vi "CPC_Surveillence_App_Overlay.vi"() -> ()   [LabVIEW 2013]
uses:
  <vilib>/userdefined/High Color/IMAQdx.ctl
  <vilib>/vision/driver/IMAQdx.llb/IMAQdx Buffer Number Mode.ctl
  <vilib>/vision/driver/NI_Vision_Acquisition_Software.lvlib
  <vilib>/vision/NI_Vision_Development_Module.lvlib
panel:
  in  "Cam1":T1
  in  "Cam0":T1
  out "Recording 2":bool
  out "Recording 2":dbl
  out "Cam 1":T2(plugin-control)
  out "Motion Detection 2":bool
  out "No Motion 2":bool caption="Time has Elapsed"
  out "Cam 0":T2(plugin-control)
  out "Motion Detection":bool
  out "No Motion":bool caption="Time has Elapsed"
  in  "Root Directory":path
  in  "Frames/s":u32=30
  out "Recording":bool
  out "Frames/s":dbl
  in  "Exit App":bool
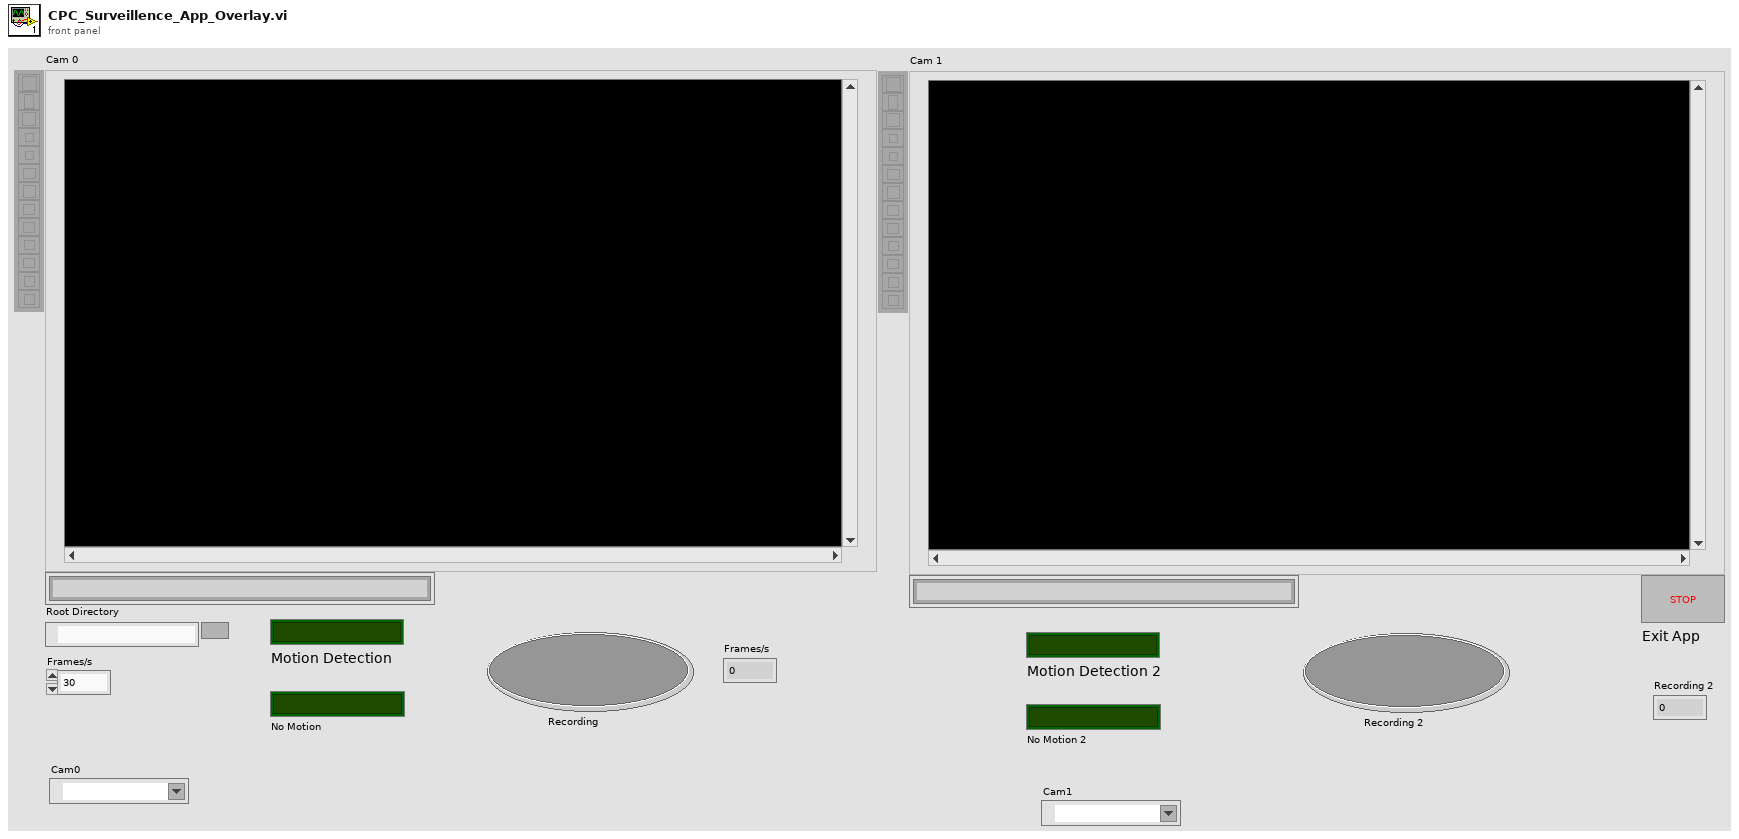
[diagram p1: front panel]
types:
  T1 = typedef "IMAQdx.ctl" = refnum<k21>
  T2 = typedef "IMAQ Image.ctl" = refnum<image>
  T3 = enum8{"Enabled", "Disabled", "Disabled and Grayed Out"}
  T4 = cluster{"Desired Font (Application)":enum16{"User-specified Font", "Application Font", "System Font", "Dialog Font"}, "[User-specified Font]":cluster{"Font Name":string, "Size":i16, "Strikeout?":bool, "Italic?":bool, "Underline?":bool, "Outline?":bool, "Shadow?":bool, "Bold?":bool, "Rotation Angle":dbl}, "Horizontal Alignment":i16, "Vertical Alignment":i16}
  T5 = typedef "NI_Vision_Acquisition_Software.lvlib/IMAQdx Buffer Number Mode.ctl" = enum32{"Next", "Last", "Buffer Number"}
  T6 = typedef "IMAQ AVI2 Refnum.ctl" = refnum<k20>
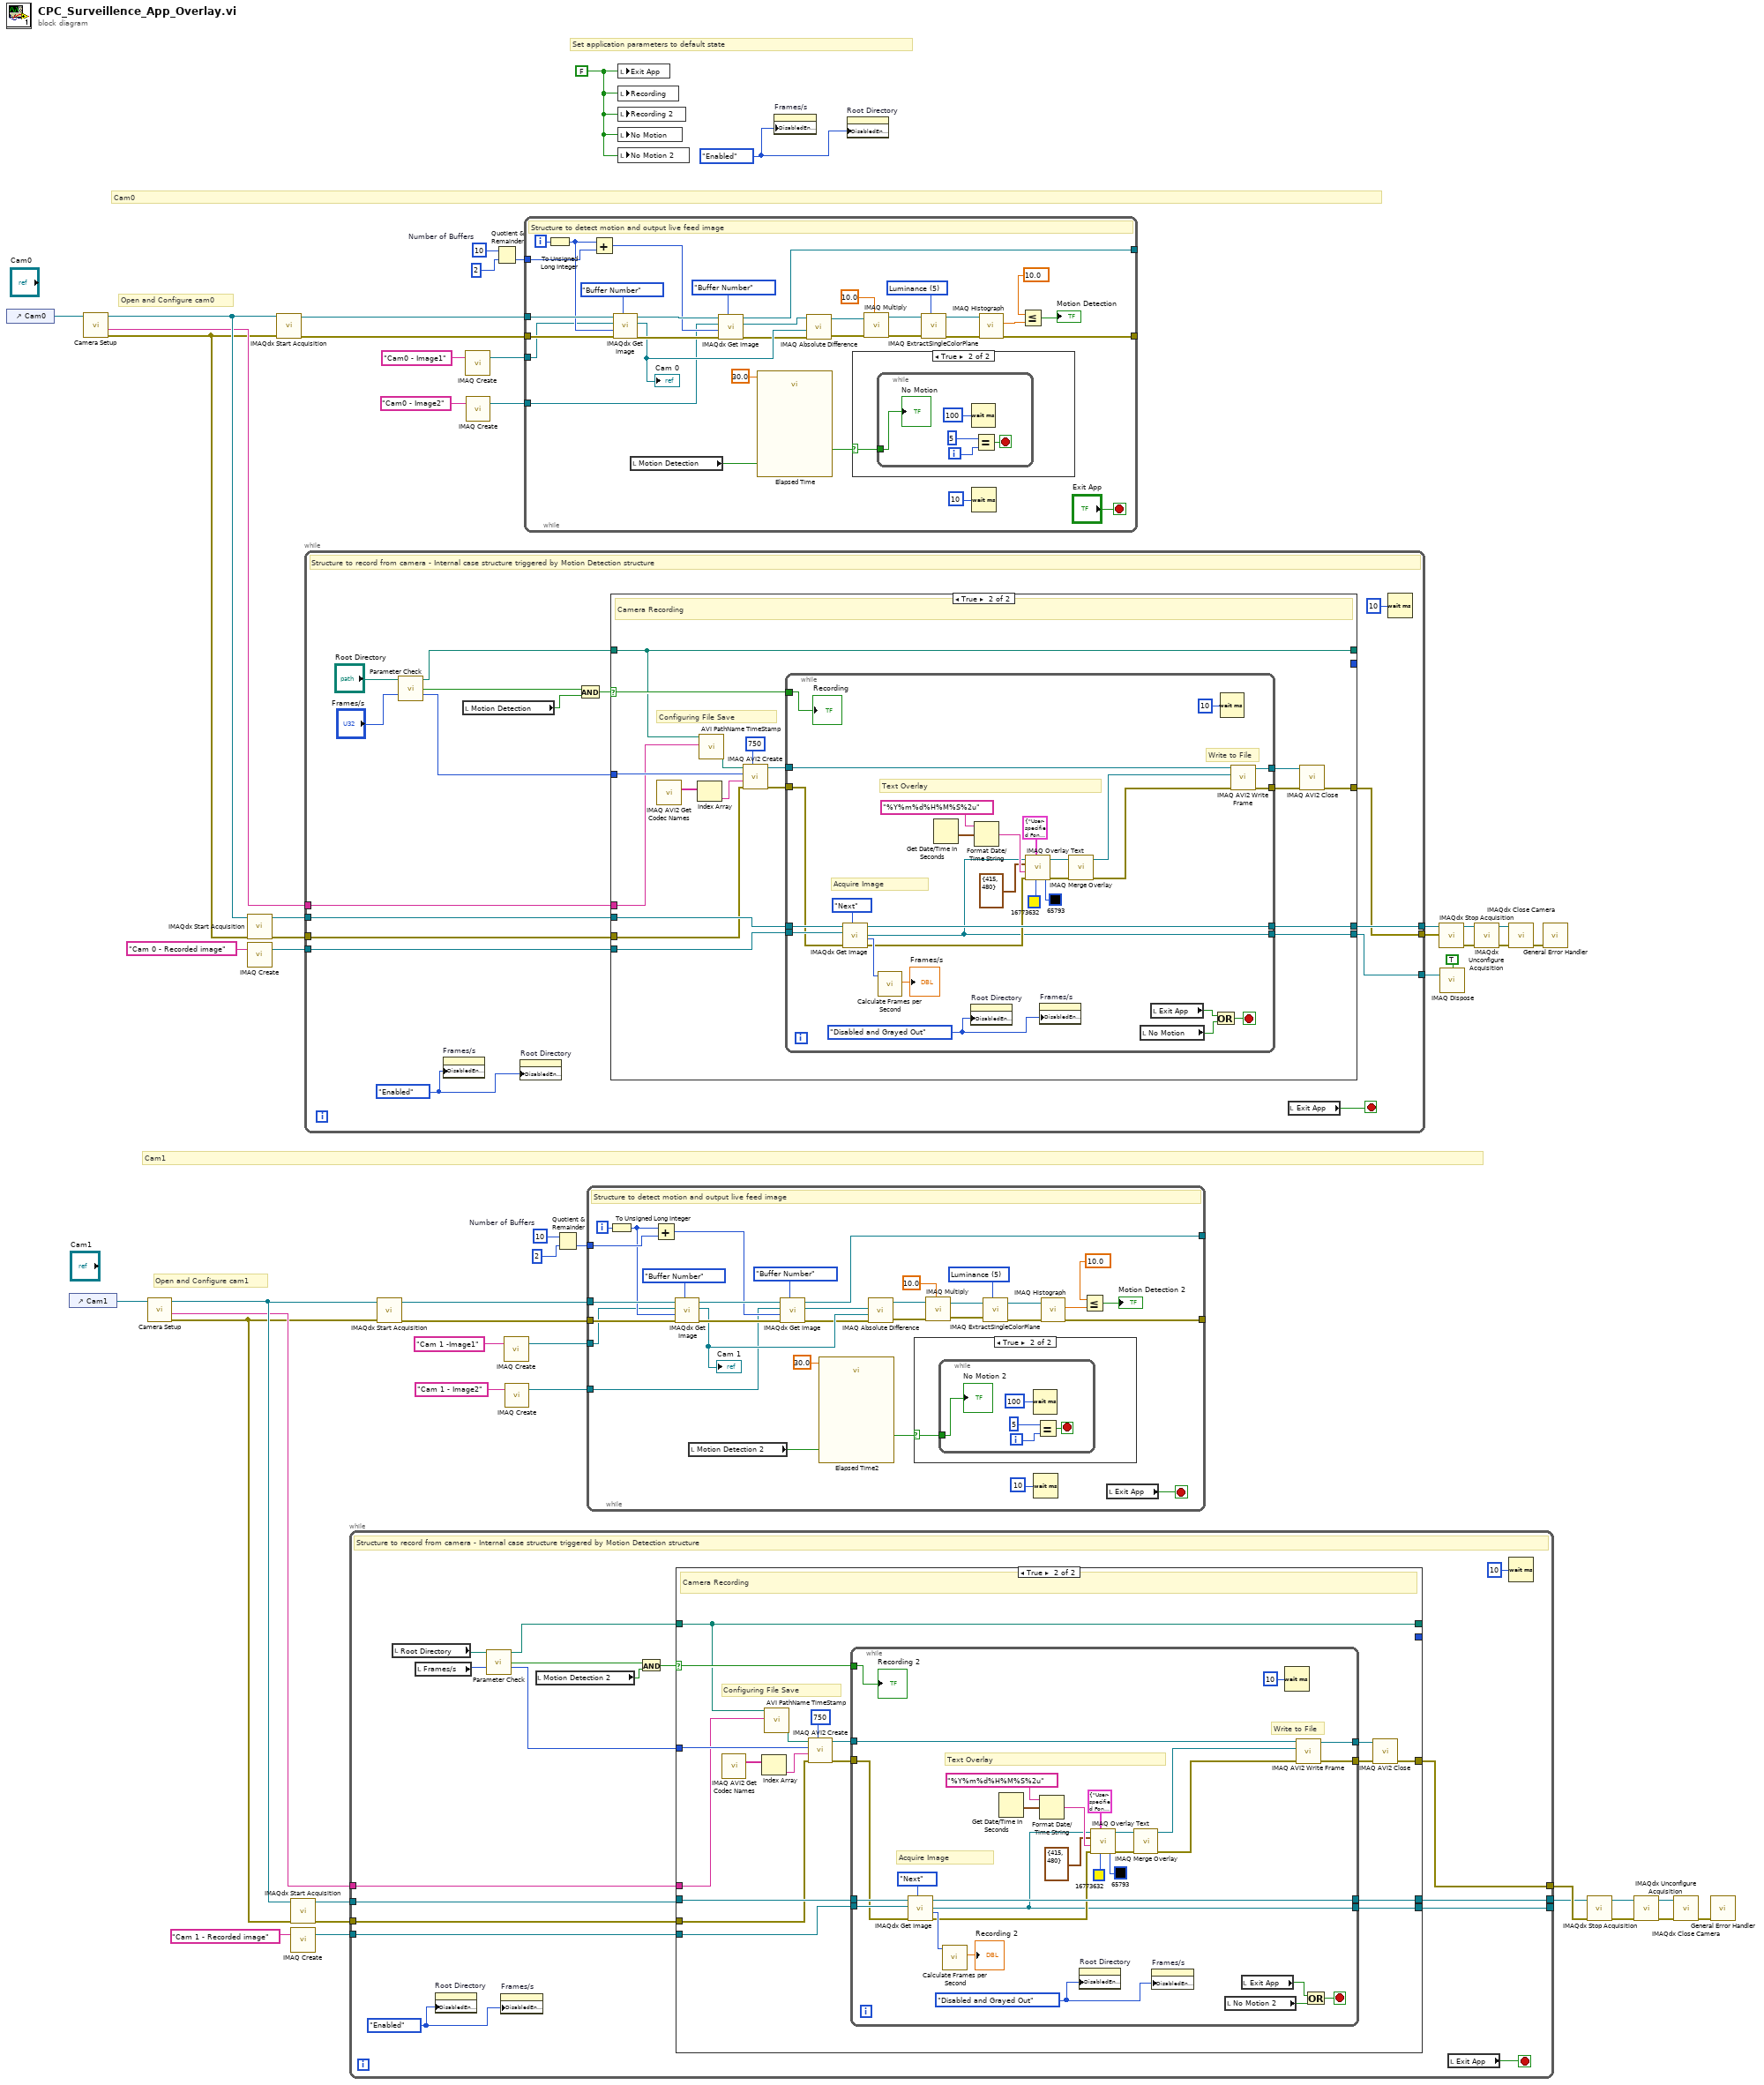
[diagram p0: block diagram]
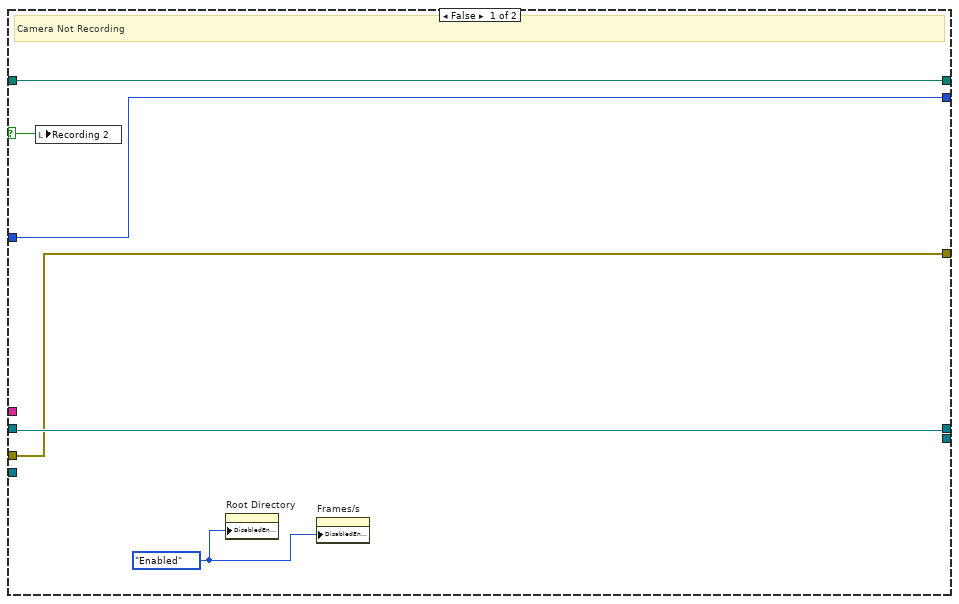
[diagram p2: hidden frame]
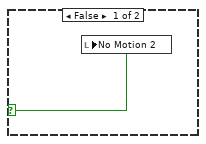
[diagram p3: hidden frame]
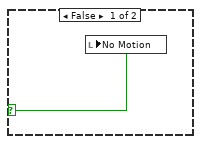
[diagram p4: hidden frame]
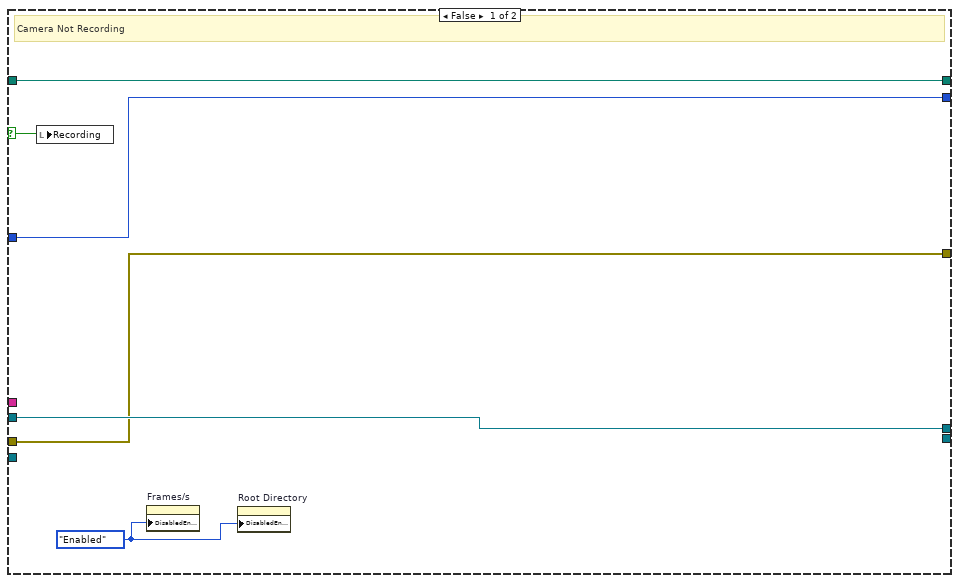
[diagram p5: hidden frame]
diagram:
  w20 = u32 10  # Number of Buffers
  w33 = u32 10  # Number of Buffers
  w36 = T3."Enabled" ("Disabled")
  w10 = FALSE ("Exit App")
  # "Cam1"
  # "Cam0"
  # "Open and Configure cam1"
  # "Open and Configure cam0"
  # "Set application parameters to default state"
  n1 = control-ref of="Cam0"() -> (w5:refnum<vi>)
  n2 = control-ref of="Cam1"() -> (w1:refnum<vi>)
  n3 = call "Camera Setup.vi"("Camera In Refnum"=w5) -> ("error out"=w6:errorcluster, "Cam Name"=w7:string, "Refnum out"=w8:T1)  [unwired: 7 in]
  n4 = call "Camera Setup.vi"("Camera In Refnum"=w1) -> ("error out"=w2:errorcluster, "Cam Name"=w3:string, "Refnum out"=w4:T1)  [unwired: 7 in]
  n5 = call <vilib>:"IMAQdx Start Acquisition.vi"("error in"=w6, "Session In"=w8) -> ("error out"=w42:errorcluster, "Session Out"=w43:T1)  [unwired: 8 in]
  n6 = call "IMAQ Create"("Image Name"="Cam 0 - Recorded image") -> ("New Image"=w44:T2)  [unwired: 3 in, 2 out]
  n7 = call <vilib>:"IMAQdx Start Acquisition.vi"("error in"=w6, "Session In"=w8) -> ("error out"=w39:errorcluster, "Session Out"=w40:T1)  [unwired: 8 out]
  n8 = call <vilib>:"IMAQdx Start Acquisition.vi"("error in"=w2, "Session In"=w4) -> ("error out"=w16:errorcluster, "Session Out"=w15:T1)  [unwired: 8 in]
  n9 = call "IMAQ Create"("Image Name"="Cam 1 - Recorded image") -> ("New Image"=w17:T2)  [unwired: 3 in, 2 out]
  n10 = while {
    tunnel: [w62] -> w18
    tunnel: [w54] -> w19
    tunnel: w42 -> [w63]
    tunnel: w43 -> [w64]
    tunnel: w44 -> [w65]
    tunnel: w7 -> [w60]
    tunnel: [w55] -> w11
    stop <- w53 stop-if-true
    w61 = T3."Enabled" ("Disabled")
    # "Structure to record from camera - Internal case structure triggered by Motion Detection structure"
    n11 = call "Parameter Check.vi"("Path"="Root Directory", "Frames Per Second in"="Frames/s") -> ("Path 2"=w56:path, "Boolean"=w59:bool, "Frames Per Second out"=w68:u32)  [unwired: 11 in]
    n12 = property on="Frames/s" class="DigNum (strict)"("DisabledEnum"=w61) -> ()  [unwired: 2 in, 2 out]
    n13 = local read "Motion Detection"() -> (w58:bool)
    n14 = property on="Root Directory" class="Path"("DisabledEnum"=w61) -> ()  [unwired: 2 in, 2 out]
    n15 = And(x=w59, y=w58) -> (x .and. y?=w57:bool)
    n16 = case shown="True" w57 {
      selector: w57 -> [w71 w81]
      tunnel: [w73 w83] -> w62
      tunnel: [w70 w82] -> w54
      tunnel: w56 -> [w75 w77]
      tunnel: w68 -> [w74 w79]
      tunnel: [w75 w77] -> _
      tunnel: [w74 _] -> _
      tunnel: w64 -> [w73 w84]
      tunnel: w63 -> [w70 w80]
      tunnel: w65 -> [_ w86]
      tunnel: w60 -> [_ w78]
      tunnel: [_ w76] -> w55
      frame False {
        w72 = T3."Enabled" ("Disabled")
        # "Camera Not Recording"
        n17 = local write "Recording"(w71) -> ()
        n18 = property on="Frames/s" class="DigNum (strict)"("DisabledEnum"=w72) -> ()  [unwired: 2 in, 2 out]
        n19 = property on="Root Directory" class="Path"("DisabledEnum"=w72) -> ()  [unwired: 2 in, 2 out]
      }
      frame True {
        # "Configuring File Save"
        # "Camera Recording"
        n20 = call "IMAQ AVI2 Get Codec Names"() -> ("Codec Names"=w89:string[])  [unwired: 10 in, 1 out]
        n21 = Index Array(array=w89) -> (element=w90:string)  [unwired: 1 in]
        n22 = call "AVI PathName TimeStamp.vi"("Root Directory"=w77, "Cam Name"=w78) -> ("appended path"=w87:path)  [unwired: 17 in]
        n23 = call "IMAQ AVI2 Create"("Quality"=750, "error in (no error)"=w80, "Codec"=w90, "Frames Per Second"=w79, "AVI Path"=w87) -> ("error out"=w85:errorcluster, "AVI Refnum"=w91:T6)  [unwired: 5 in]
        n24 = while {
          tunnel: w84 -> [w119]
          tunnel: w85 -> [w107]
          tunnel: w86 -> [w121]
          tunnel: [w104] -> w83
          tunnel: w91 -> [w118]
          tunnel: [w117] -> w92
          tunnel: [w116] -> w82
          tunnel: w81 -> [w110]
          tunnel: [w96] -> w76
          stop <- w111 stop-if-true
          w114 = T3."Disabled and Grayed Out" ("Disabled")
          # "Write to File"
          # "Acquire Image"
          # "Text Overlay"
          n25 = call <vilib>:"IMAQdx Get Image.vi"("Buffer Number Mode (Next)"=IMAQdx_Buffer_Number_Mode."Next", "error in"=w107, "Image In"=w121, "Session In"=w119) -> ("error out"=w102:errorcluster, "Buffer Number Out"=w109:u32, "Image Out"=w96:T2, "Session Out"=w104:T1)  [unwired: 4 in]
          n26 = call <vilib>:"Calculate Frames per Second.vi"("Buffer Number"=w109) -> ("Processed Frames/s"=→"Frames/s":dbl)  [unwired: 8 in, 2 out]
          n27 = Get Date/Time In Seconds() -> (seconds since 1Jan1904=w105:timestamp)
          n28 = property on="Root Directory" class="Path"("DisabledEnum"=w114) -> ()  [unwired: 2 in, 2 out]
          n29 = Format Date/Time String(time format string (%c)="%Y%m%d%H%M%S%2u", seconds (now)=w105) -> (date/time string=w103:string)  [unwired: 1 in]
          n30 = call "IMAQ Overlay Text"("BG Color (Transparent)"=u32 65793, "Text Color (black)"=u32 16773632, "Font, Size & Style"=T4 {"Desired Font (Application)"=enum."User-specified Font", "[User-specified Font]"={"Font Name"="", "Size"=24, "Strikeout?"=FALSE, "Italic?"=FALSE, "Underline?"=FALSE, "Outline?"=FALSE, "Shadow?"=FALSE, "Bold?"=FALSE, "Rotation Angle"=0.0}, "Horizontal Alignment"=0, "Vertical Alignment"=0}, "error in (no error)"=w102, "String"=w103, "Origin"=cluster{"X":i32, "Y":i32} {"X"=415, "Y"=480}, "Image"=w96) -> ("error out"=w99:errorcluster, "Image Out"=w100:T2)  [unwired: 3 in]
          n31 = property on="Frames/s" class="DigNum (strict)"("DisabledEnum"=w114) -> ()  [unwired: 2 in, 2 out]
          n32 = call "IMAQ Merge Overlay"("error in (no error)"=w99, "Image Src"=w100) -> ("error out"=w97:errorcluster, "Image Dst Out"=w98:T2)  [unwired: 8 in]
          n33 = local read "No Motion"() -> (w112:bool)
          n34 = local read "Exit App"() -> (w113:bool)
          n35 = Or(x=w113, y=w112) -> (x .or. y?=w111:bool)
          n36 = Wait (ms)(milliseconds to wait=u32 10) -> ()  [unwired: 1 out]
          n37 = call "IMAQ AVI2 Write Frame"("error in (no error)"=w97, "Image"=w98, "AVI Refnum"=w118) -> ("error out"=w116:errorcluster, "AVI Refnum (duplicate)"=w117:T6)  [unwired: 6 in, 1 out]
          "Recording" <- w110
        }
        n38 = call "IMAQ AVI2 Close"("error in (no error)"=w82, "AVI Refnum"=w92) -> ()  [unwired: 9 in, 1 out]
      }
    }
    n39 = local read "Exit App"() -> (w53:bool)
    n40 = Wait (ms)(milliseconds to wait=u32 10) -> ()  [unwired: 1 out]
  }
  n41 = while {
    tunnel: [w126] -> w9
    tunnel: [w125] -> w14
    tunnel: w16 -> [w129]
    tunnel: w15 -> [w124]
    tunnel: [w127] -> _
    tunnel: w17 -> [w128]
    tunnel: w3 -> [w130]
    stop <- w136 stop-if-true
    w122 = T3."Enabled" ("Disabled")
    # "Structure to record from camera - Internal case structure triggered by Motion Detection structure"
    n42 = local read "Root Directory"() -> (w135:path)
    n43 = local read "Frames/s"() -> (w134:u32)
    n44 = property on="Root Directory" class="Path"("DisabledEnum"=w122) -> ()  [unwired: 2 in, 2 out]
    n45 = call "Parameter Check.vi"("Path"=w135, "Frames Per Second in"=w134) -> ("Path 2"=w132:path, "Boolean"=w137:bool, "Frames Per Second out"=w123:u32)  [unwired: 11 in]
    n46 = property on="Frames/s" class="DigNum (strict)"("DisabledEnum"=w122) -> ()  [unwired: 2 in, 2 out]
    n47 = local read "Motion Detection 2"() -> (w133:bool)
    n48 = And(x=w137, y=w133) -> (x .and. y?=w131:bool)
    n49 = case shown="True" w131 {
      selector: w131 -> [w139 w150]
      tunnel: [w142 w152] -> w126
      tunnel: [w141 w151] -> w125
      tunnel: w132 -> [w144 w146]
      tunnel: w123 -> [w143 w148]
      tunnel: [w144 w146] -> _
      tunnel: [w143 _] -> _
      tunnel: w124 -> [w142 w153]
      tunnel: w129 -> [w141 w149]
      tunnel: w128 -> [_ w155]
      tunnel: w130 -> [_ w147]
      tunnel: [_ w145] -> w127
      frame False {
        w140 = T3."Enabled" ("Disabled")
        # "Camera Not Recording"
        n50 = local write "Recording 2"(w139) -> ()
        n51 = property on="Root Directory" class="Path"("DisabledEnum"=w140) -> ()  [unwired: 2 in, 2 out]
        n52 = property on="Frames/s" class="DigNum (strict)"("DisabledEnum"=w140) -> ()  [unwired: 2 in, 2 out]
      }
      frame True {
        # "Configuring File Save"
        # "Camera Recording"
        n53 = call "IMAQ AVI2 Get Codec Names"() -> ("Codec Names"=w158:string[])  [unwired: 10 in, 1 out]
        n54 = Index Array(array=w158) -> (element=w159:string)  [unwired: 1 in]
        n55 = call "AVI PathName TimeStamp.vi"("Root Directory"=w146, "Cam Name"=w147) -> ("appended path"=w156:path)  [unwired: 17 in]
        n56 = call "IMAQ AVI2 Create"("Quality"=750, "error in (no error)"=w149, "Codec"=w159, "Frames Per Second"=w148, "AVI Path"=w156) -> ("error out"=w154:errorcluster, "AVI Refnum"=w160:T6)  [unwired: 5 in]
        n57 = while {
          tunnel: w153 -> [w188]
          tunnel: w154 -> [w179]
          tunnel: w155 -> [w190]
          tunnel: [w176] -> w152
          tunnel: w160 -> [w187]
          tunnel: [w186] -> w161
          tunnel: [w185] -> w151
          tunnel: w150 -> [w182]
          tunnel: [w168] -> w145
          stop <- w183 stop-if-true
          w162 = T3."Disabled and Grayed Out" ("Disabled")
          # "Write to File"
          # "Acquire Image"
          # "Text Overlay"
          n58 = call <vilib>:"IMAQdx Get Image.vi"("Buffer Number Mode (Next)"=IMAQdx_Buffer_Number_Mode."Next", "error in"=w179, "Image In"=w190, "Session In"=w188) -> ("error out"=w174:errorcluster, "Buffer Number Out"=w181:u32, "Image Out"=w168:T2, "Session Out"=w176:T1)  [unwired: 4 in]
          n59 = call <vilib>:"Calculate Frames per Second.vi"("Buffer Number"=w181) -> ("Processed Frames/s"=→"Recording 2":dbl)  [unwired: 8 in, 2 out]
          n60 = Get Date/Time In Seconds() -> (seconds since 1Jan1904=w177:timestamp)
          n61 = Format Date/Time String(time format string (%c)="%Y%m%d%H%M%S%2u", seconds (now)=w177) -> (date/time string=w175:string)  [unwired: 1 in]
          n62 = property on="Root Directory" class="Path"("DisabledEnum"=w162) -> ()  [unwired: 2 in, 2 out]
          n63 = call "IMAQ Overlay Text"("BG Color (Transparent)"=u32 65793, "Text Color (black)"=u32 16773632, "Font, Size & Style"=T4 {"Desired Font (Application)"=enum."User-specified Font", "[User-specified Font]"={"Font Name"="", "Size"=24, "Strikeout?"=FALSE, "Italic?"=FALSE, "Underline?"=FALSE, "Outline?"=FALSE, "Shadow?"=FALSE, "Bold?"=FALSE, "Rotation Angle"=0.0}, "Horizontal Alignment"=0, "Vertical Alignment"=0}, "error in (no error)"=w174, "String"=w175, "Origin"=cluster{"X":i32, "Y":i32} {"X"=415, "Y"=480}, "Image"=w168) -> ("error out"=w171:errorcluster, "Image Out"=w172:T2)  [unwired: 3 in]
          n64 = call "IMAQ Merge Overlay"("error in (no error)"=w171, "Image Src"=w172) -> ("error out"=w169:errorcluster, "Image Dst Out"=w170:T2)  [unwired: 8 in]
          n65 = property on="Frames/s" class="DigNum (strict)"("DisabledEnum"=w162) -> ()  [unwired: 2 in, 2 out]
          n66 = local read "No Motion 2"() -> (w164:bool)
          n67 = local read "Exit App"() -> (w163:bool)
          n68 = Wait (ms)(milliseconds to wait=u32 10) -> ()  [unwired: 1 out]
          n69 = call "IMAQ AVI2 Write Frame"("error in (no error)"=w169, "Image"=w170, "AVI Refnum"=w187) -> ("error out"=w185:errorcluster, "AVI Refnum (duplicate)"=w186:T6)  [unwired: 6 in, 1 out]
          n70 = Or(x=w163, y=w164) -> (x .or. y?=w183:bool)
          "Recording 2" <- w182
        }
        n71 = call "IMAQ AVI2 Close"("error in (no error)"=w151, "AVI Refnum"=w161) -> ()  [unwired: 9 in, 1 out]
      }
    }
    n72 = local read "Exit App"() -> (w136:bool)
    n73 = Wait (ms)(milliseconds to wait=u32 10) -> ()  [unwired: 1 out]
  }
  n74 = call <vilib>:"IMAQdx Start Acquisition.vi"("error in"=w2, "Session In"=w4) -> ("error out"=w23:errorcluster, "Session Out"=w24:T1)  [unwired: 8 out]
  n75 = call "IMAQ Create"("Image Name"="Cam0 - Image1") -> ("New Image"=w48:T2)  [unwired: 3 in, 2 out]
  n76 = call "IMAQ Create"("Image Name"="Cam0 - Image2") -> ("New Image"=w46:T2)  [unwired: 3 in, 2 out]
  n77 = Quotient & Remainder(x=w33, y=u32 2) -> (floor(x/y)=w34:u32)  [unwired: 1 out]
  n78 = call "IMAQ Create"("Image Name"="Cam 1 -Image1") -> ("New Image"=w28:T2)  [unwired: 3 in, 2 out]
  n79 = call "IMAQ Create"("Image Name"="Cam 1 - Image2") -> ("New Image"=w26:T2)  [unwired: 3 in, 2 out]
  n80 = while {
    tunnel: w48 -> [w204]
    tunnel: w40 -> [w221]
    tunnel: w39 -> [w222]
    tunnel: w46 -> [w203]
    tunnel: [w216] -> _
    tunnel: [w205] -> _
    tunnel: w34 -> [w210]
    i -> [w209]
    stop <- "Exit App" stop-if-true
    w196 = 5 items=["Red", "Green", "Blue", "Hue", "Saturation", "Luminance", "Value", "Intensity"] ("Color Plane")
    # "Structure to detect motion and output live feed image"
    n81 = To Unsigned Long Integer(number=w209) -> (unsigned 32bit integer=w208:u32)
    n82 = Add(x=w208, y=w210) -> (x+y=w211:u32)
    n83 = call <vilib>:"IMAQdx Get Image.vi"("Buffer Number Mode (Next)"=IMAQdx_Buffer_Number_Mode."Buffer Number", "error in"=w222, "Buffer Number In"=w208, "Image In"=w204, "Session In"=w221) -> ("error out"=w218:errorcluster, "Image Out"=w212:T2, "Session Out"=w217:T1)  [unwired: 4 out]
    "Cam 0" <- w212
    n84 = local read "Motion Detection"() -> (w193:bool)
    n85 = call <vilib>:"IMAQdx Get Image.vi"("Buffer Number Mode (Next)"=IMAQdx_Buffer_Number_Mode."Buffer Number", "error in"=w218, "Buffer Number In"=w211, "Image In"=w203, "Session In"=w217) -> ("error out"=w206:errorcluster, "Image Out"=w215:T2, "Session Out"=w216:T1)  [unwired: 4 out]
    n86 = call "Elapsed Time"("Time Target (s)"=30.0, "Reset"=w193) -> ("Time has Elapsed"=w192:bool)  [unwired: 10 in, 7 out]
    n87 = call "IMAQ Absolute Difference"("Image Src A"=w215, "Image Src B"=w212, "error in (no error)"=w206) -> ("Image Dst Out"=w214:T2, "error out"=w207:errorcluster)  [unwired: 2 in, 2 out]
    n88 = case shown="True" w192 {
      selector: w192 -> [w224 w225]
      frame False {
        n89 = local write "No Motion"(w224) -> ()
      }
      frame True {
        n90 = while {
          tunnel: w225 -> [w226]
          i -> [w228]
          stop <- w227 stop-if-true
          n91 = Wait (ms)(milliseconds to wait=u32 100) -> ()  [unwired: 1 out]
          n92 = Equal?(x=5, y=w228) -> (x = y?=w227:bool)
          "No Motion" <- w226
        }
      }
    }
    n93 = call "IMAQ Multiply"("Image Src A"=w214, "Constant"=sgl 10.0 ("Pixel Gain"), "error in (no error)"=w207) -> ("Image Dst Out"=w200:T2, "error out"=w199:errorcluster)  [unwired: 2 in, 2 out]
    n94 = call "IMAQ ExtractSingleColorPlane"("Color Plane"=w196, "error in (no error)"=w199, "Image Src"=w200) -> ("error out"=w197:errorcluster, "Image Dst Out"=w198:T2)  [unwired: 7 in]
    n95 = Wait (ms)(milliseconds to wait=u32 10) -> ()  [unwired: 1 out]
    n96 = call "IMAQ Histograph"("error in (no error)"=w197, "Image"=w198) -> ("error out"=w205:errorcluster, "Mean Value"=w201:sgl)  [unwired: 3 in, 5 out]
    n97 = Less Or Equal?(x=sgl 10.0 ("Mean Pixel Value Threshold"), y=w201) -> (x <= y?=→"Motion Detection":bool)
  }
  n98 = Quotient & Remainder(x=w20, y=u32 2) -> (floor(x/y)=w21:u32)  [unwired: 1 out]
  n99 = while {
    tunnel: w28 -> [w244]
    tunnel: w24 -> [w261]
    tunnel: w23 -> [w262]
    tunnel: w26 -> [w243]
    tunnel: [w256] -> _
    tunnel: [w245] -> _
    tunnel: w21 -> [w250]
    i -> [w249]
    stop <- w232 stop-if-true
    w236 = 5 items=["Red", "Green", "Blue", "Hue", "Saturation", "Luminance", "Value", "Intensity"] ("Color Plane")
    # "Structure to detect motion and output live feed image"
    n100 = To Unsigned Long Integer(number=w249) -> (unsigned 32bit integer=w248:u32)
    n101 = Add(x=w248, y=w250) -> (x+y=w251:u32)
    n102 = call <vilib>:"IMAQdx Get Image.vi"("Buffer Number Mode (Next)"=IMAQdx_Buffer_Number_Mode."Buffer Number", "error in"=w262, "Buffer Number In"=w248, "Image In"=w244, "Session In"=w261) -> ("error out"=w258:errorcluster, "Image Out"=w252:T2, "Session Out"=w257:T1)  [unwired: 4 out]
    "Cam 1" <- w252
    n103 = local read "Motion Detection 2"() -> (w234:bool)
    n104 = call <vilib>:"IMAQdx Get Image.vi"("Buffer Number Mode (Next)"=IMAQdx_Buffer_Number_Mode."Buffer Number", "error in"=w258, "Buffer Number In"=w251, "Image In"=w243, "Session In"=w257) -> ("error out"=w246:errorcluster, "Image Out"=w255:T2, "Session Out"=w256:T1)  [unwired: 4 out]
    n105 = call "Elapsed Time2"("Time Target (s)"=30.0, "Reset"=w234) -> ("Time has Elapsed"=w233:bool)  [unwired: 10 in, 7 out]
    n106 = call "IMAQ Absolute Difference"("Image Src A"=w255, "Image Src B"=w252, "error in (no error)"=w246) -> ("Image Dst Out"=w254:T2, "error out"=w247:errorcluster)  [unwired: 2 in, 2 out]
    n107 = case shown="True" w233 {
      selector: w233 -> [w264 w265]
      frame False {
        n108 = local write "No Motion 2"(w264) -> ()
      }
      frame True {
        n109 = while {
          tunnel: w265 -> [w266]
          i -> [w268]
          stop <- w267 stop-if-true
          n110 = Wait (ms)(milliseconds to wait=u32 100) -> ()  [unwired: 1 out]
          n111 = Equal?(x=5, y=w268) -> (x = y?=w267:bool)
          "No Motion 2" <- w266
        }
      }
    }
    n112 = call "IMAQ Multiply"("Image Src A"=w254, "Constant"=sgl 10.0 ("Pixel Gain"), "error in (no error)"=w247) -> ("Image Dst Out"=w240:T2, "error out"=w239:errorcluster)  [unwired: 2 in, 2 out]
    n113 = call "IMAQ ExtractSingleColorPlane"("Color Plane"=w236, "error in (no error)"=w239, "Image Src"=w240) -> ("error out"=w237:errorcluster, "Image Dst Out"=w238:T2)  [unwired: 7 in]
    n114 = Wait (ms)(milliseconds to wait=u32 10) -> ()  [unwired: 1 out]
    n115 = call "IMAQ Histograph"("error in (no error)"=w237, "Image"=w238) -> ("error out"=w245:errorcluster, "Mean Value"=w241:sgl)  [unwired: 3 in, 5 out]
    n116 = Less Or Equal?(x=sgl 10.0 ("Mean Pixel Value Threshold"), y=w241) -> (x <= y?=→"Motion Detection 2":bool)
    n117 = local read "Exit App"() -> (w232:bool)
  }
  n118 = local write "Exit App"(w10) -> ()
  n119 = local write "Recording"(w10) -> ()
  n120 = local write "Recording 2"(w10) -> ()
  n121 = local write "No Motion"(w10) -> ()
  n122 = local write "No Motion 2"(w10) -> ()
  n123 = property on="Frames/s" class="DigNum (strict)"("DisabledEnum"=w36) -> ()  [unwired: 2 in, 2 out]
  n124 = property on="Root Directory" class="Path"("DisabledEnum"=w36) -> ()  [unwired: 2 in, 2 out]
  n125 = call <vilib>:"IMAQdx Stop Acquisition.vi"("error in"=w19, "Session In"=w18) -> ("error out"=w38:errorcluster, "Session Out"=w41:T1)  [unwired: 8 in]
  n126 = call "IMAQ Dispose"("All Images? (No)"=TRUE, "Image"=w11) -> ()  [unwired: 4 in, 1 out]
  n127 = call <vilib>:"IMAQdx Unconfigure Acquisition.vi"("error in"=w38, "Session In"=w41) -> ("error out"=w52:errorcluster, "Session Out"=w50:T1)  [unwired: 8 in]
  n128 = call <vilib>:"IMAQdx Close Camera.vi"("error in"=w52, "Session In"=w50) -> ("error out"=w51:errorcluster)  [unwired: 9 in]
  n129 = call <vilib>:"General Error Handler.vi"("error in (no error)"=w51) -> ()  [unwired: 1 in, 14 out]
  n130 = call <vilib>:"IMAQdx Stop Acquisition.vi"("error in"=w14, "Session In"=w9) -> ("error out"=w13:errorcluster, "Session Out"=w12:T1)  [unwired: 8 in]
  n131 = call <vilib>:"IMAQdx Unconfigure Acquisition.vi"("error in"=w13, "Session In"=w12) -> ("error out"=w32:errorcluster, "Session Out"=w30:T1)  [unwired: 8 in]
  n132 = call <vilib>:"IMAQdx Close Camera.vi"("error in"=w32, "Session In"=w30) -> ("error out"=w31:errorcluster)  [unwired: 9 in]
  n133 = call <vilib>:"General Error Handler.vi"("error in (no error)"=w31) -> ()  [unwired: 1 in, 14 out]
